vi "Error Handler.vi"(8 "error in (no error)":errorcluster, 11 "Enum in":T1=enum."Initalization") -> (0 "error out":errorcluster, 3 "Enum out":T1=enum."Initalization")   [LabVIEW 2015]
uses:
  Cases.ctl
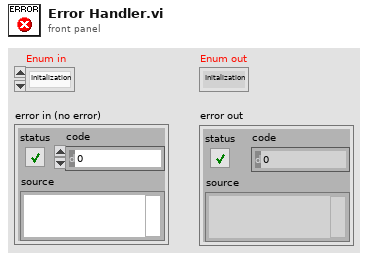
[diagram p1: front panel]
types:
  T1 = typedef "Cases.ctl" = enum16{"Start", "Initalization", "J16 Test", "J15 Test", "J15 Error Page", "K2 Test", "K2 Error Page", "K3 Test", "K3 Error Page", "K4 Test", "K4 Error Page", "Test Complete", "Test Failed", "Error", "J15 Failed", "J16 Error", "J16 Failed", "K2 Failed", "LEDs Failed"}
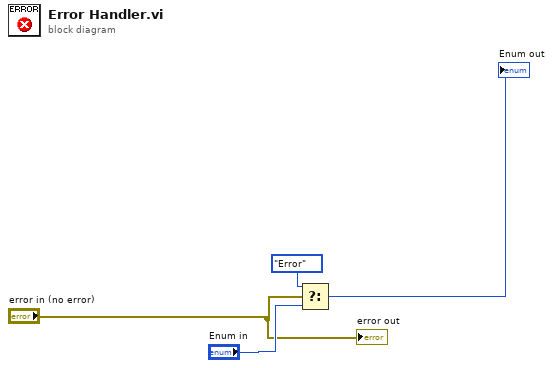
[diagram p0: block diagram]
diagram:
  n1 = Select(t=Cases."Error" ("Enum"), s="error in (no error)", f="Enum in") -> (s? t:f=→"Enum out":T1)
  "error out" <- "error in (no error)"
